vi "Connect (Dynamic).vi"(5 "SqlMapper":string(combo)="ado", 7 "DbType":string(combo)="Npgsql", 8 "error in (no error)":errorcluster, 11 "Connection String":string) -> (0 "error out":errorcluster, 3 "SqlMapper out":refnum<class "SqlMapper.lvclass">)   [LabVIEW 2020, in "ORM_API.lvlib"]
uses:
  ORM_API.lvlib
  <vilib>/Viviota/shared/ORM.lvlibp/ORM/SqlMapper/SqlMapper.lvclass
  <vilib>/Viviota/shared/ORM.lvlibp/ORM/DbConnection/DbConnection.lvclass
  <vilib>/Utility/LVLibp/NI_PackedLibraryUtility.lvlib
panel:
  # "to add quotes to SQLite table names\ninclude:\n\nORMQuotesOnTableName=true|false;"
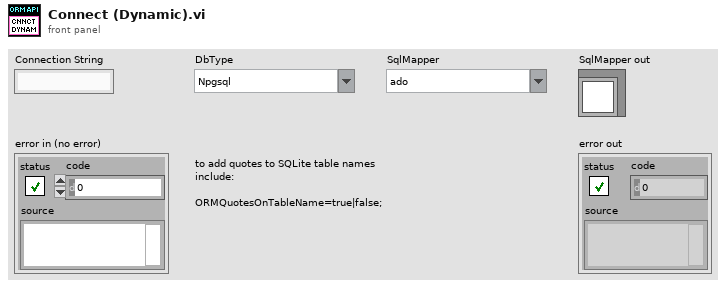
[diagram p1: front panel]
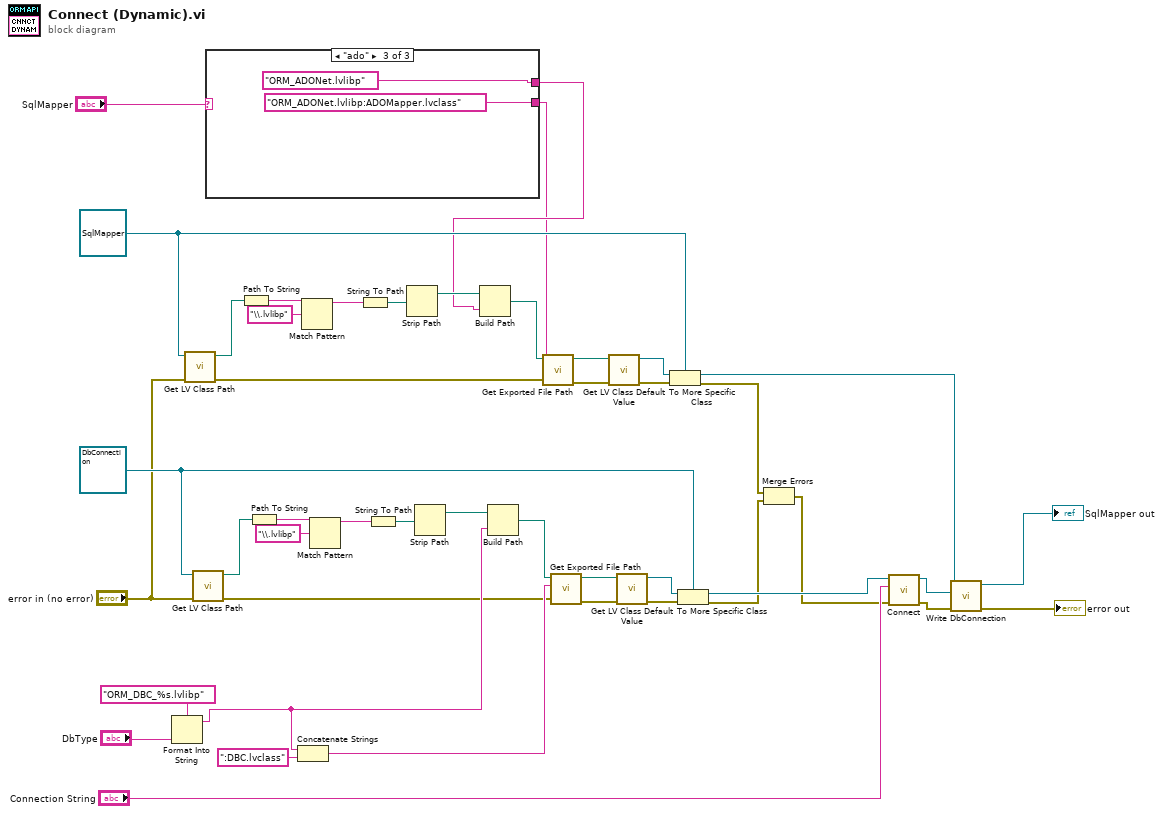
[diagram p0: block diagram]
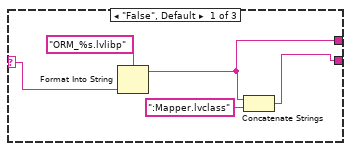
[diagram p2: hidden frame]
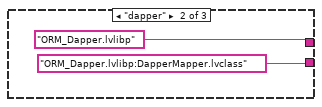
[diagram p3: hidden frame]
diagram:
  w8 = refnum<class "SqlMapper.lvclass"> refnum ("Type In")
  w25 = refnum<class "DbConnection.lvclass"> refnum ("Dapper.lvlib:DbConnection.lvclass")
  n1 = Format Into String(format string="ORM_DBC_%s.lvlibp", "DbType") -> (resulting string=w33:string)  [unwired: 2 in, 1 out]
  n2 = call <vilib>:"Get LV Class Path.vi"("error in (no error)"="error in (no error)", "object"=w8) -> ("error out"=w17:errorcluster, "class path"=w10:path)  [unwired: 8 in]
  n3 = call <vilib>:"Get LV Class Path.vi"("error in (no error)"="error in (no error)", "object"=w25) -> ("error out"=w30:errorcluster, "class path"=w42:path)  [unwired: 8 in]
  n4 = case shown="\"ado\"" "SqlMapper" {
    selector: "SqlMapper" -> [w48 _ _]
    tunnel: [w47 "ORM_Dapper.lvlibp:DapperMapper.lvclass" "ORM_ADONet.lvlibp:ADOMapper.lvclass"] -> w5
    tunnel: [w46 "ORM_Dapper.lvlibp" "ORM_ADONet.lvlibp"] -> w6
    frame "False", Default {
      n5 = Format Into String(format string="ORM_%s.lvlibp", w48) -> (resulting string=w46:string)  [unwired: 2 in, 1 out]
      n6 = Concatenate Strings(w46, ":Mapper.lvclass" ("string")) -> (w47:string)
    }
    frame "dapper" {
    }
    frame "ado" {
    }
  }
  n7 = Path To String(path=w10) -> (string=w11:string)
  n8 = Path To String(path=w42) -> (string=w41:string)
  n9 = Concatenate Strings(w33, ":DBC.lvclass" ("string")) -> (w31:string)
  n10 = Match Pattern(string=w11, regular expression="\\.lvlibp") -> (before substring=w13:string)  [unwired: 1 in, 3 out]
  n11 = Match Pattern(string=w41, regular expression="\\.lvlibp") -> (before substring=w39:string)  [unwired: 1 in, 3 out]
  n12 = String To Path(string=w13) -> (path=w14:path)
  n13 = String To Path(string=w39) -> (path=w38:path)
  n14 = Strip Path(path=w14) -> (stripped path=w15:path)  [unwired: 1 out]
  n15 = Strip Path(path=w38) -> (stripped path=w35:path)  [unwired: 1 out]
  n16 = Build Path(base path=w15, name or relative path=w6) -> (appended path=w16:path)
  n17 = Build Path(base path=w35, name or relative path=w33) -> (appended path=w34:path)
  n18 = call <vilib>:"Get Exported File Path.vi"("error in (no error)"=w17, "qualified name"=w5, "packed library path"=w16) -> ("error out"=w18:errorcluster, "path"=w20:path)  [unwired: 7 in]
  n19 = call <vilib>:"Get Exported File Path.vi"("error in (no error)"=w30, "qualified name"=w31, "packed library path"=w34) -> ("error out"=w29:errorcluster, "path"=w27:path)  [unwired: 7 in]
  n20 = call <vilib>:"Get LV Class Default Value.vi"("error in (no error)"=w18, "class path"=w20) -> ("error out"=w19:errorcluster, "object"=w21:refnum<class>)  [unwired: 8 in]
  n21 = call <vilib>:"Get LV Class Default Value.vi"("error in (no error)"=w29, "class path"=w27) -> ("error out"=w28:errorcluster, "object"=w26:refnum<class>)  [unwired: 8 in]
  n22 = To More Specific Class(target class=w8, reference=w21, error in=w19) -> (specific class reference=w4:refnum<class "SqlMapper.lvclass">, error out=w3:errorcluster)
  n23 = To More Specific Class(target class=w25, reference=w26, error in=w28) -> (specific class reference=w24:refnum<class "DbConnection.lvclass">, error out=w2:errorcluster)
  n24 = Merge Errors(w3, w2) -> (w1:errorcluster)
  n25 = call-dynamic "Connect.vi"("error in (no error)"=w1, "Connection String"="Connection String", "DbConnection Type"=w24) -> ("error out"=w23:errorcluster, "DbConnection out"=w43:refnum<class "DbConnection.lvclass">)  [unwired: 7 in]
  n26 = call <vilib>:"Write DbConnection.vi"("error in (no error)"=w23, "Dapper.lvlib:DbConnection.lvclass"=w43, "SqlMapper in"=w4) -> ("error out"=→"error out":errorcluster, "SqlMapper out"=→"SqlMapper out":refnum<class "SqlMapper.lvclass">)  [unwired: 7 in]
